vi "Table Value To 1D I32 Without Exception Number.vi"(8 "End Number":i32, 9 "Exception Number":i32=-1, 11 "Table Ref In":refnum<vi>) -> (1 "I32 Out":i32[](array[numeric]), 3 "Table Ref Out":refnum<vi>)   [LabVIEW 2024]
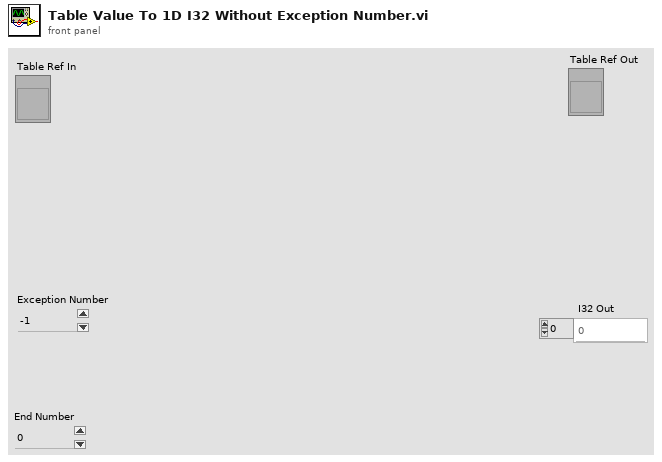
[diagram p1: front panel]
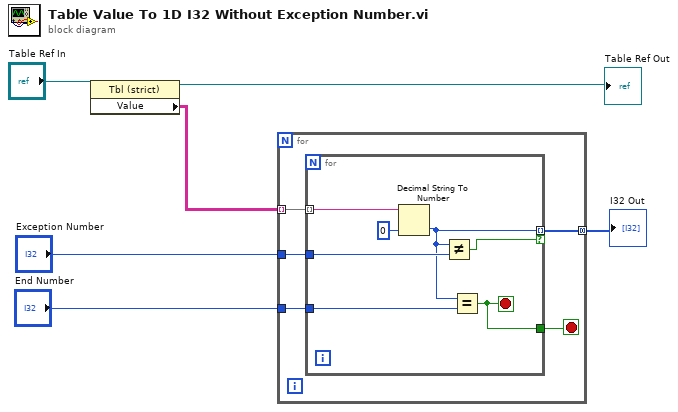
[diagram p0: block diagram]
diagram:
  n1 = property class="Tbl (strict)"(reference="Table Ref In") -> (reference out=→"Table Ref Out":refnum<vi>, "Value"=w4:string[][])  [unwired: 1 in, 1 out]
  n2 = for {
    tunnel: w4 -> [w11] mode=indexing
    tunnel: "Exception Number" -> [w10]
    tunnel: [w9] -> w2 mode=concatenating
    tunnel: "End Number" -> [w8]
    stop <- w7 stop-if-true
    n3 = for {
      tunnel: w11 -> [w18] mode=indexing
      tunnel: [w13] -> w9 mode=indexing if=w16
      tunnel: w10 -> [w15]
      tunnel: w8 -> [w14]
      tunnel: [w12] -> w7
      stop <- w12 stop-if-true
      n4 = Decimal String To Number(string=w18, default (0L)=0 ("default (0 I32)")) -> (number=w13:i32)  [unwired: 1 in, 1 out]
      n5 = Not Equal?(x=w13, y=w15) -> (x != y?=w16:bool)
      n6 = Equal?(x=w13, y=w14) -> (x = y?=w12:bool)
    }
  }
  "I32 Out" <- w2
